vi "3_AdvancedDemo_HHT3.vi"() -> ()   [LabVIEW 2020]
uses:
  Types/HH_InputChannel.ctl
  Types/HH_UIThread_Cmds.ctl
  Types/HH_UIThread_Data.ctl
  _lib/PQ/HydraHarp/HH_InitInfo.ctl
  Types/HH_DataProcThread_QData.ctl
  Types/HH_DataProcThread_QCmds.ctl
  Types/HH_VisThread_QData.ctl
  Types/HH_VisThread_QCmds.ctl
  Types/HH_VisThread_Data.ctl
  _lib/PQ/HydraHarp/HH_RefSource.ctl
  _lib/PQ/HydraHarp/HH_MeasMode.ctl
  <vilib>/Utility/error.llb/DialogType.ctl
  _lib/PQ/HydraHarp/hhlib_x86_x64_UIThread.llb/HH_DllPath_global.vi
  <vilib>/Utility/error.llb/Error Cluster From Error Code.vi
  _lib/PQ/HydraHarp/HH_LibVersion_global.vi
  <vilib>/ErrorRing/Error Ring.xnode
panel:
  in  "Settings":bool=TRUE
  in  "Run continuously":bool caption="Conti."
  in  "Start":bool
  in  "Scale":bool
  out "CountRates":i32[](graph)
  in  "HistoAcqTime":dbl=1.0 caption="Int.Time    s" min=0.1 max=360000.0 step=0.1
  in  "AcqTime":i32=360000000 caption="T3Acq.   ms" min=1 max=360000 step=1
  in  "Binning":i32(ring) caption="Resol.      ps" items=["1", "2", "4", "8", "16", "32", "64", "128", "256", "512", "1024", "2048", "4096", "8192", "16384", "32768", "65536", "131072", "262144", "524288", "1048576", "2097152", "4194304", "8388608", "16777216", "33554432"]
  in  "HistoOffset":i32 caption="Offset      ns" min=0 max=500000 step=1
  out "DeltaT":dbl=inf caption="Resol.     ms" format="%.2f"
  in  "BitShift":i32=15 min=0 max=32 step=1
  in  "OvlLevel":i32=65536 caption="Ovl.Level" min=1024 max=65536 step=1024
  in  "StopOvl.":bool=TRUE
  out "TTraceGraph":T1(graph)
  out "HistoGraph":cluster{dbl, "Resol":dbl, "Histos":u32[][]}(graph)
  in  "SyncZeroX":i32=10 caption="ZeroCr.  mV" min=0 max=40 step=1
  in  "SyncDivider":i32(ring)=3 caption="Divider" items=["1", "2", "4", "8", "16"]
  in  "SyncOffset":i32 caption="Offset      ps" min=-99999 max=99999 step=1
  in  "SyncLevel":i32=50 caption="Level      mV" min=0 max=1000 step=1
  in  "Channels":T2[](array[typedef])=[{"Name"="Inp.Chan 1", "Enable"=TRUE, "Offset"=0, "CFDLevel"=50, "ZeroX"=10}, {"Name"="Inp.Chan 2", "Enable"=TRUE, "Offset"=0, "CFDLevel"=50, "ZeroX"=10}, {"Name"="Inp.Chan 3", "Enable"=TRUE, "Offset"=0, "CFDLevel"=50, "ZeroX"=10}, {"Name"="Inp.Chan 4", "Enable"=TRUE, "Offset"=0, "CFDLevel"=50, "ZeroX"=10}, {"Name"="Inp.Chan 5", "Enable"=TRUE, "Offset"=0, "CFDLevel"=50, "ZeroX"=10}, {"Name"="Inp.Chan 6", "Enable"=TRUE, "Offset"=0, "CFDLevel"=50, "ZeroX"=10}, {"Name"="Inp.Chan 7", "Enable"=TRUE, "Offset"=0, "CFDLevel"=50, "ZeroX"=10}, {"Name"="Inp.Chan 8", "Enable"=TRUE, "Offset"=0, "CFDLevel"=50, "ZeroX"=10}] {"ZeroX" min=0 max=40 step=1; "Offset" min=-99999 max=99999 step=1; "CFDLevel" min=0 max=1000 step=1}
  out "SyncRate":string="Sync Rate: 0 cps\n"
  out "OverRun":bool caption="Overrun:"
  out "Status":string="Elements in Q: 0"
  # "Histogram"
  # "Time Trace"
  # "Sync"
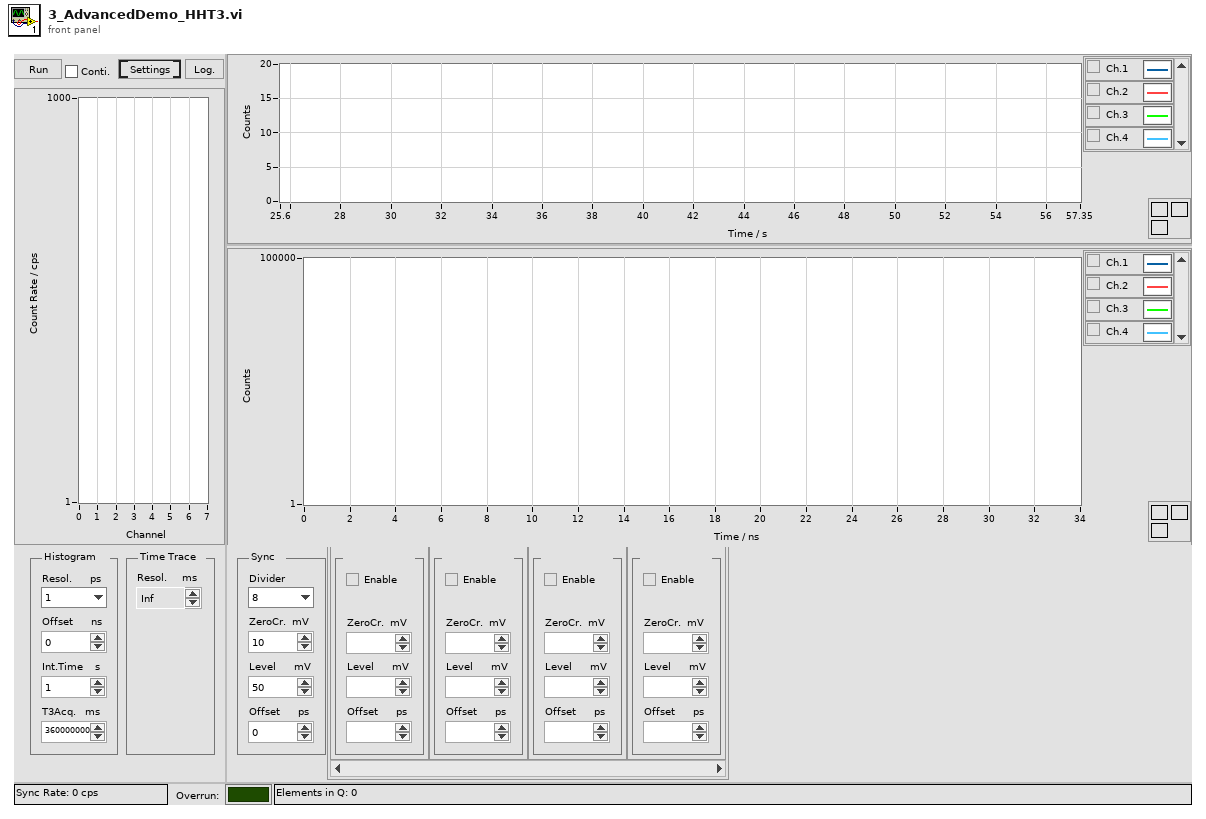
[diagram p1: front panel]
types:
  T1 = cluster{dbl, "Resolution":dbl, "Histogram":u32[][]}
  T2 = typedef "HH_InputChannel.ctl" = cluster{"Name":string, "Enable":bool, "Offset":i32, "CFDLevel":i32, "ZeroX":i32}
  T3 = typedef "HH_DataProcThread_QCmds.ctl" = enum16{"Exit", "Proc", "Init", "SetShift", "SetNumChannels", "SetHistAcqTime"}
  T4 = typedef "HH_VisThread_Data.ctl" = cluster{"Resol":dbl, "DeltaT":dbl, "NumChannels":i32}
  T5 = typedef "HH_VisThread_QData.ctl" = cluster{"Histos":u32[][], "Cmd":T6, "TimeTrace":u32[][], "Bin":i32, "Total bin":u64, "Status":string, "Resol":dbl, "DeltaT":dbl, "nChannels":i32}
  T6 = typedef "HH_VisThread_QCmds.ctl" = enum16{"_none_", "Resol", "nChannels", "DeltaT", "Histo", "TTrace", "Status"}
  T7 = typedef "HH_DataProcThread_QData.ctl" = cluster{"Cmd":T3, "nActual":i32, "Buffer":u32[], "TickCount":u32, "Param":i32}
  T8 = typedef "HH_UIThread_Data.ctl" = cluster{"Init Info":T9, "DevIdx":i32, "SyncDivider":i32, "SyncOffset":i32, "SyncLevel":i32, "Channels":T2[], "CurrentChannels":i32[], "AcqTime":i32, "Binning":i32, "HistoOffset":i32, "HistoLen":i32, "StopOvl.":bool, "OvlLevel":u32, "StartMeas":bool, "HistoLength":i32, "Resolution":dbl, "Run cont.":bool, "Status":string, "SyncRate":i32, "BitShift":i32, "HistoAcqTime":dbl, "SyncZeroX":i32, "SyncRateStart":i32}
  T9 = typedef "HH_InitInfo.ctl" = cluster{"Library Version":string, "Serial No.":string, "Model":string, "Partnum":string, "Version":string, "features":i32, "nchannels":i32, "nummod":i32, "Model Codes":i32[], "Version Codes":i32[], "Base Resolution":dbl, "Bin Steps":i32}
  T10 = typedef "HH_UIThread_Cmds.ctl" = enum16{"Idle", "Init", "SetInpChanEnable", "SetInpChanOffset", "SetInpChanTrg", "SetSyncDivider", "SetSyncTrg", "SetSyncOffset", "SetBinning", "SetHistoOffset", "SetHistoLen", "SetStopOvl", "SetBitShift", "SetHistoAcqTime", "GetRates", "StartMeas", "StopMeas", "AbortMeas", "GetResolution", "GetHisto", "ReadFiFo", "WriteStatus", "Resize", "EnableControls", "DisableControls", "Error", "Exit"}
  T11 = enum8{"Enabled", "Disabled", "Disabled and Grayed Out"}
  T12 = typedef "HH_MeasMode.ctl" = i32
  T13 = typedef "HH_RefSource.ctl" = enum16{"internal", "external"}
  T14 = typedef "DialogType.ctl" = u16
  T15 = cluster{"T0":dbl, "dt":dbl, "TimeTrace_out":u32[][]}
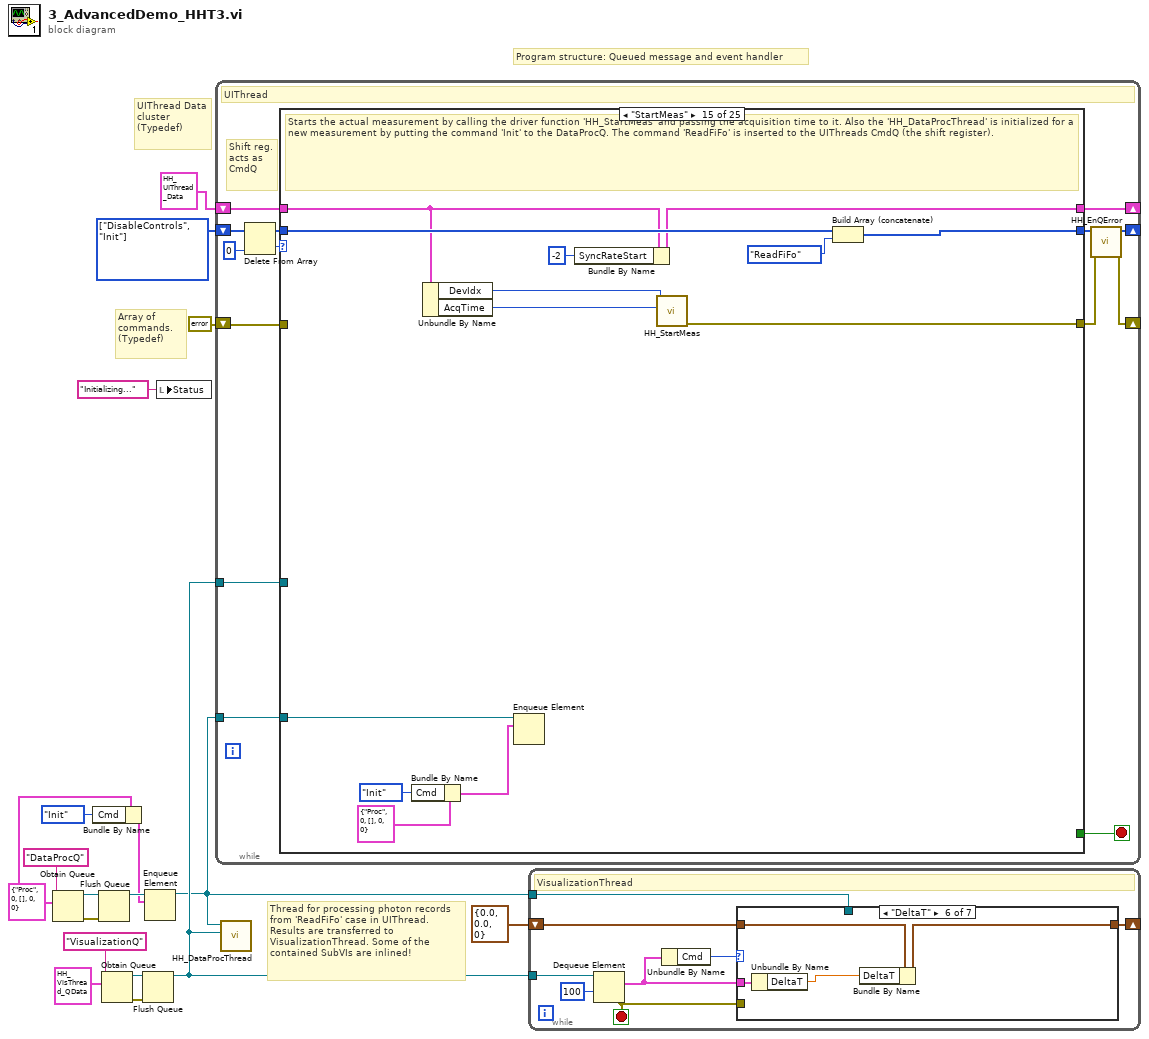
[diagram p0: block diagram]
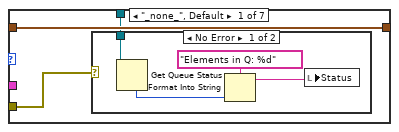
[diagram p2: hidden frame]
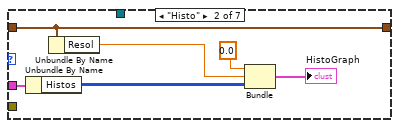
[diagram p4: hidden frame]
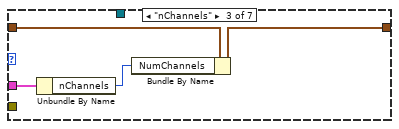
[diagram p5: hidden frame]
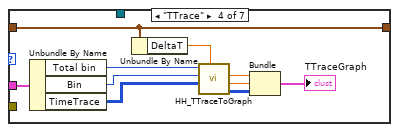
[diagram p6: hidden frame]
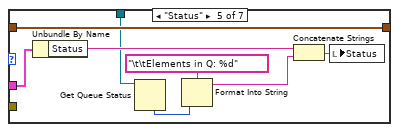
[diagram p7: hidden frame]
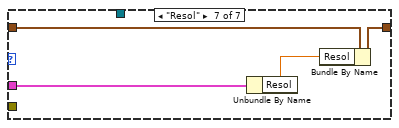
[diagram p8: hidden frame]
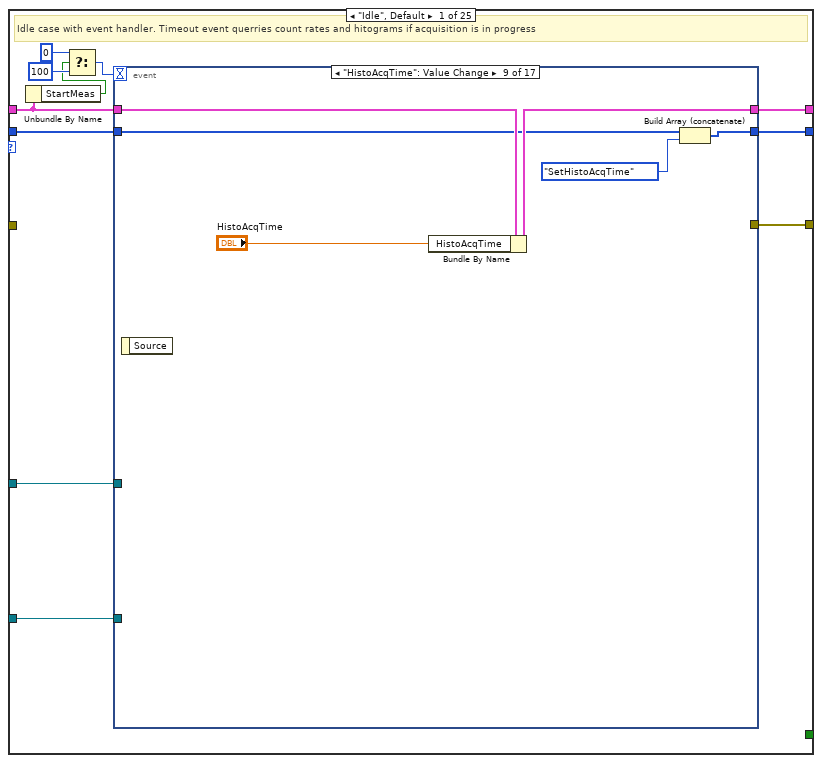
[diagram p9: hidden frame]
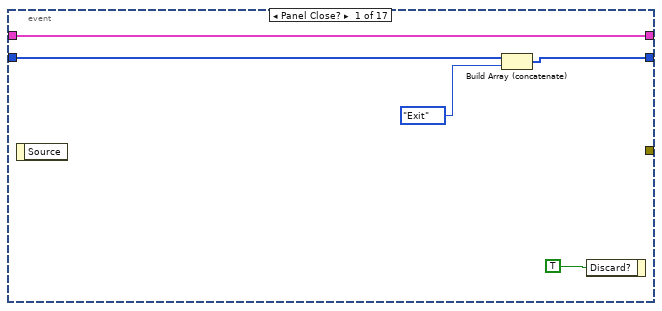
[diagram p10: hidden frame]
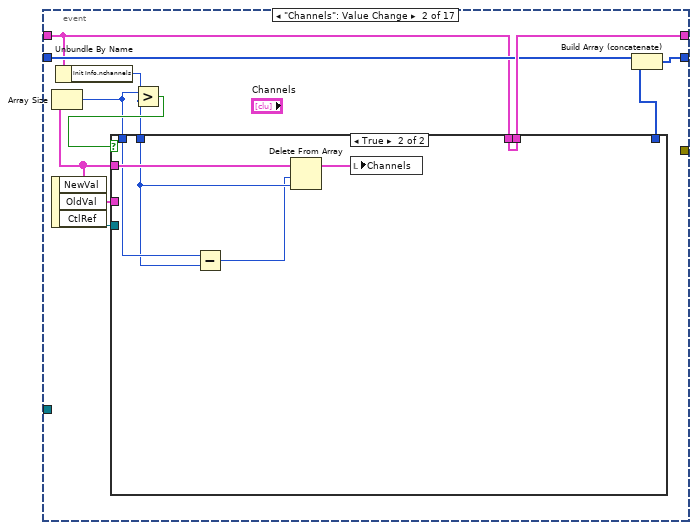
[diagram p11: hidden frame]
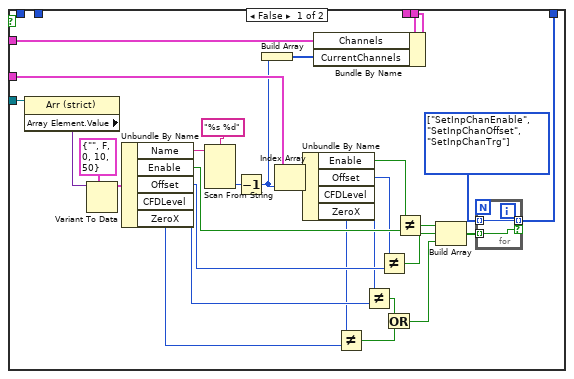
[diagram p12: hidden frame]
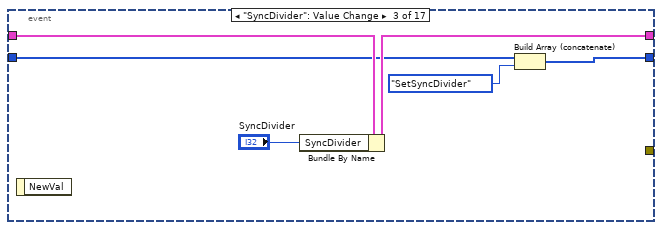
[diagram p13: hidden frame]
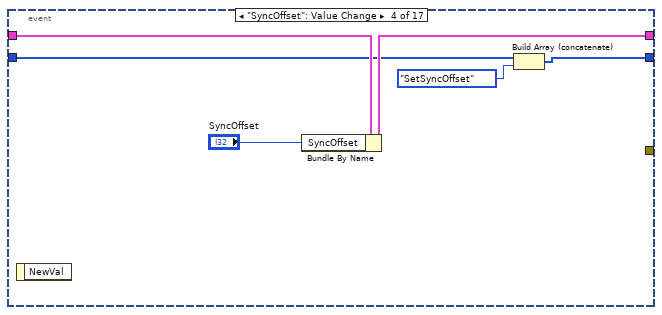
[diagram p14: hidden frame]
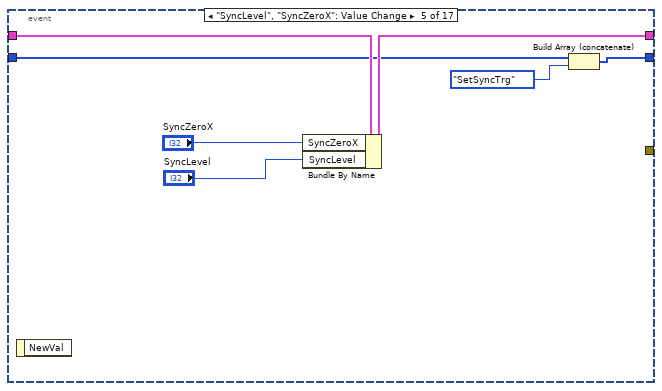
[diagram p15: hidden frame]
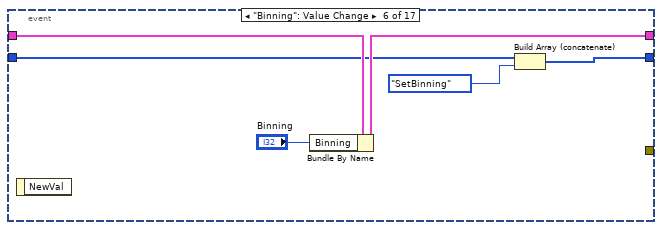
[diagram p16: hidden frame]
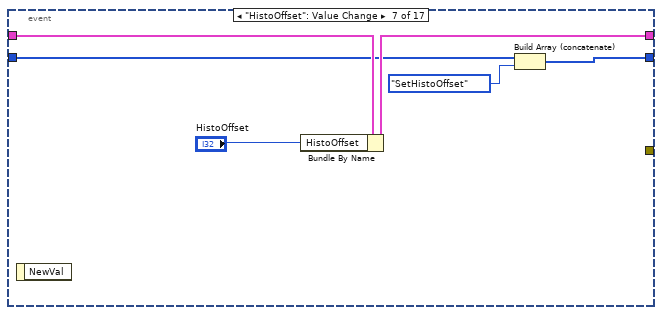
[diagram p17: hidden frame]
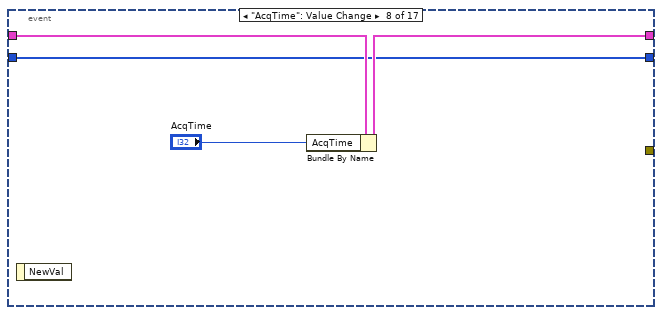
[diagram p18: hidden frame]
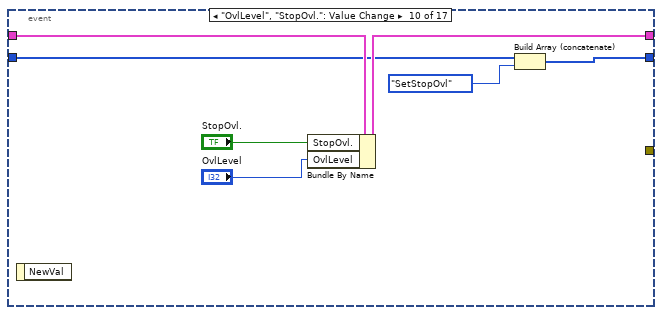
[diagram p19: hidden frame]
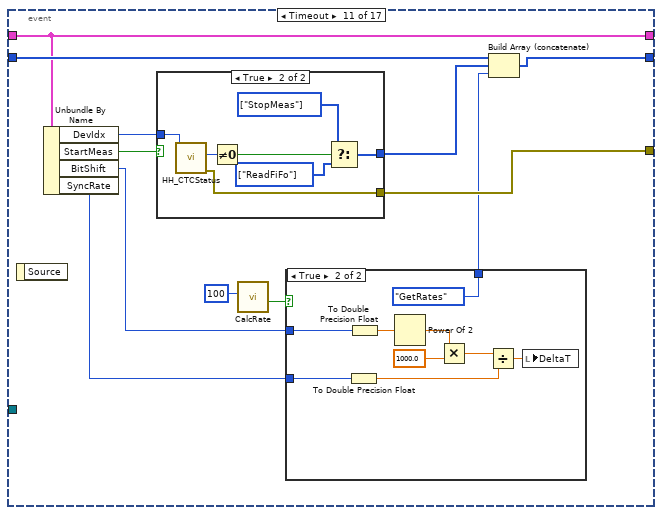
[diagram p20: hidden frame]
diagram:
  w4 = T7 {"Cmd"=enum."Proc", "nActual"=0, "Buffer"=[], "TickCount"=0, "Param"=0} ("MH_DataProcThread_QData")
  w17 = T10[] [enum."DisableControls", enum."Init"] items=["Idle", "Init", "SetInpChanEnable", "SetInpChanOffset", "SetInpChanTrg", "SetSyncDivider", "SetSyncTrg", "SetSyncOffset", "SetBinning", "SetHistoOffset", "SetHistoLen", "SetStopOvl", "SetBitShift", "SetHistoAcqTime", "GetRates", "StartMeas", "StopMeas", "AbortMeas", "GetResolution", "GetHisto", "ReadFiFo", "WriteStatus", "Resize", "EnableControls", "DisableControls", "Error", "Exit"]
  # "Thread for processing photon records from 'ReadFiFo' case in UIThread. Results are transferred to VisualizationThread. Some of the contained SubVIs are inlined!"
  # "Array of commands.\n(Typedef)"
  # "Program structure: Queued message and event handler"
  # "UIThread Data cluster\n(Typedef)"
  n1 = Obtain Queue(name (unnamed)="DataProcQ", element data type=w4) -> (queue out=w14:refnum<queue>, error out=w13:errorcluster)  [unwired: 3 in, 1 out]
  n2 = Bundle By Name(cluster=w4, "Cmd"=HH_DataProcThread_QCmds."Init") -> (w2:T7)
  n3 = Flush Queue(queue=w14, error in (no error)=w13) -> (queue out=w5:refnum<queue>)  [unwired: 2 out]
  n4 = Obtain Queue(name (unnamed)="VisualizationQ", element data type=T5 {"Histos"=[], "Cmd"=enum."_none_", "TimeTrace"=[], "Bin"=0, "Total bin"=0, "Status"="", "Resol"=0.0, "DeltaT"=0.0, "nChannels"=0} ("MH_GUIThread_QData")) -> (queue out=w12:refnum<queue>, error out=w11:errorcluster)  [unwired: 3 in, 1 out]
  n5 = Flush Queue(queue=w12, error in (no error)=w11) -> (queue out=w7:refnum<queue>)  [unwired: 2 out]
  n6 = Enqueue Element(queue=w5, element=w2) -> (queue out=w1:refnum<queue>)  [unwired: 2 in, 2 out]
  n7 = local write "Status"("Initializing..." ("Status")) -> ()
  n8 = while {
    shift-right: [w21] -> _
    shift-left: w17 -> [w28]
    shift-right: [w31] -> _
    shift-left: T8 {"Init Info"={"Library Version"="", "Serial No."="", "Model"="", "Partnum"="", "Version"="", "features"=0, "nchannels"=0, "nummod"=0, "Model Codes"=[], "Version Codes"=[], "Base Resolution"=0.0, "Bin Steps"=0}, "DevIdx"=0, "SyncDivider"=1, "SyncOffset"=0, "SyncLevel"=50, "Channels"=[], "CurrentChannels"=[], "AcqTime"=1, "Binning"=1, "HistoOffset"=1, "HistoLen"=1024, "StopOvl."=FALSE, "OvlLevel"=1024, "StartMeas"=FALSE, "HistoLength"=0, "Resolution"=0.0, "Run cont."=FALSE, "Status"="", "SyncRate"=0, "BitShift"=0, "HistoAcqTime"=0.0, "SyncZeroX"=10, "SyncRateStart"=0} -> [w30]
    shift-right: [w23] -> _
    shift-left: errorcluster {"status"=FALSE, "code"=0, "source"=""} ("error IO") -> [w29]
    tunnel: w1 -> [w20]
    tunnel: w7 -> [w19]
    stop <- w32 stop-if-true
    # "Shift reg.\nacts as\nCmdQ"
    # "UIThread"
    n9 = Delete From Array(array=w28, index=0) -> (deleted portion=w26:T10, array with subset deleted=w25:T10[])  [unwired: 1 in]
    n10 = case shown="\"StartMeas\"" w26 {
      tunnel: [w43 w272 w301 w315 w329 w346 w355 w357 w364 w372 w379 w399 w411 w420 w498 w503 w516 w533 w534 w560 w573 w580 w592 w598 w604] -> w22
      tunnel: [_ _ _ _ _ _ _ _ _ _ _ _ _ _ _ _ _ _ _ _ _ _ _ _ TRUE] -> w32
      tunnel: [w42 w253 w304 w318 w332 w348 w356 w361 w368 w373 w380 w384 w401 w423 w490 w506 w518 w529 w544 w559 w561 w579 w591 w599 w607] -> w31
      tunnel: w30 -> [w39 w258 w304 w318 w332 w348 w356 w361 w368 w373 w380 w384 w401 w419 w491 w507 w519 w530 w544 w559 w561 w579 w591 w599 w607]
      tunnel: [w40 w277 w302 w316 w330 w344 w354 w360 w367 w371 w378 _ _ w429 w501 w509 w521 w531 w539 _ _ _ _ _ w605] -> w24
      tunnel: w29 -> [_ _ _ _ _ _ _ _ _ _ _ _ _ _ _ _ _ _ _ _ _ _ _ w600 _]
      tunnel: w25 -> [w41 w274 w301 w315 w329 w346 w355 w357 w363 w372 w379 w399 w411 w421 w499 w504 w516 w533 w535 w560 w573 w580 w592 _ w604]
      tunnel: w20 -> [w34 w251 _ _ _ _ _ _ _ _ _ w385 w402 _ w495 _ _ _ w536 _ _ _ _ _ w603]
      tunnel: w19 -> [w33 w243 _ _ _ _ _ _ _ _ _ w386 _ _ _ _ _ w526 _ _ _ _ _ _ w602]
      frame "Idle", Default {
        # "Idle case with event handler. Timeout event querries count rates and hitograms if acquisition is in progress"
        n11 = Unbundle By Name(w39) -> ("StartMeas"=w37:bool)
        n12 = Select(t=0, s=w37, f=100) -> (s? t:f=w36:i32)
        n13 = event shown="[8] \"HistoAcqTime\": Value Change" {
          selector: _ -> [_ _ _ _ _ _ _ _ _ _ _ _ _ _ _ _ _]
          dyn-events: _ -> [_ _ _ _ _ _ _ _ _ _ _ _ _ _ _ _ _]
          timeout: w36 -> [_ _ _ _ _ _ _ _ _ _ _ _ _ _ _ _ _]
          tunnel: [w44 w54 w98 w104 w111 w118 w124 w129 w134 w141 w156 w174 w186 w204 w210 w218 w228] -> w43
          tunnel: [w47 w57 w102 w108 w115 w121 w127 w131 w137 w144 w155 w178 w185 w202 w209 w217 w231] -> w42
          tunnel: w39 -> [w47 w53 w103 w109 w116 w122 w128 w132 w138 w145 w155 w179 w183 w203 w209 w217 w231]
          tunnel: w41 -> [w46 w56 w100 w106 w113 w120 w126 w129 w135 w143 w157 w175 w187 w204 w210 w218 w229]
          tunnel: [_ _ _ _ _ _ _ _ _ _ w151 _ _ _ _ _ _] -> w40
          tunnel: w34 -> [_ _ _ _ _ _ _ _ _ _ _ _ _ _ _ _ _]
          tunnel: w33 -> [_ _ _ _ _ _ _ _ _ _ _ _ _ _ _ _ _]
          event Panel Close? {
            n14 = event-data() -> ()  [unwired: 1 in, 1 out]
            n15 = Build Array (concatenate)(w46, HH_UIThread_Cmds."Exit") -> (w44:T10[])
            n16 = event-data("Discard?"=TRUE) -> ()  [unwired: 1 in, 1 out]
          }
          event "Channels": Value Change {
            n17 = event-data() -> ("NewVal"=w52:T2[], "OldVal"=w58:T2[], "CtlRef"=w59:refnum<vi>)  [unwired: 1 in]
            n18 = Array Size(array=w52) -> (size(s)=w49:i32)
            n19 = Unbundle By Name(w53) -> ("Init Info.nchannels"=w50:i32)
            n20 = Greater?(x=w49, y=w50) -> (0:w51:bool)
            n21 = case shown="True" w51 {
              tunnel: w59 -> [w89 _]
              tunnel: w58 -> [w83 _]
              tunnel: [w66 w97] -> w57
              tunnel: [w64 _] -> w55
              tunnel: w53 -> [w61 w97]
              tunnel: w52 -> [w60 w96]
              tunnel: w50 -> [_ w94]
              tunnel: w49 -> [_ w95]
              frame False {
                w67 = T10[] [enum."SetInpChanEnable", enum."SetInpChanOffset", enum."SetInpChanTrg"] items=["Idle", "Init", "SetInpChanEnable", "SetInpChanOffset", "SetInpChanTrg", "SetSyncDivider", "SetSyncTrg", "SetSyncOffset", "SetBinning", "SetHistoOffset", "SetHistoLen", "SetStopOvl", "SetBitShift", "SetHistoAcqTime", "GetRates", "StartMeas", "StopMeas", "AbortMeas", "GetResolution", "GetHisto", "ReadFiFo", "WriteStatus", "Resize", "EnableControls", "DisableControls", "Error", "Exit"]
                n22 = property class="Arr (strict)"(reference=w89) -> ("Array Element.Value"=w88:variant)  [unwired: 1 in, 2 out]
                n23 = Variant To Data(type=T2 {"Name"="", "Enable"=FALSE, "Offset"=0, "CFDLevel"=10, "ZeroX"=50} ("Channel"), Variant=w88) -> (data=w65:T2)  [unwired: 1 in, 1 out]
                n24 = Unbundle By Name(w65) -> ("Name"=w86:string, "Enable"=w80:bool, "Offset"=w78:i32, "CFDLevel"=w76:i32, "ZeroX"=w74:i32)
                n25 = Scan From String(format string="%s %d", input string=w86) -> (output 2=w84:i32)  [unwired: 5 in, 3 out]
                n26 = Decrement(x=w84) -> (x-1=w63:i32)
                n27 = Build Array(w63) -> (w62:i32[])
                n28 = Index Array(array=w83, index=w63) -> (element=w82:T2)
                n29 = Unbundle By Name(w82) -> ("Enable"=w81:bool, "Offset"=w79:i32, "CFDLevel"=w77:i32, "ZeroX"=w75:i32)
                n30 = Bundle By Name(cluster=w61, "Channels"=w60, "CurrentChannels"=w62) -> (w66:T8)
                n31 = Not Equal?(x=w75, y=w74) -> (x != y?=w69:bool)
                n32 = Not Equal?(x=w77, y=w76) -> (x != y?=w70:bool)
                n33 = Not Equal?(x=w79, y=w78) -> (x != y?=w72:bool)
                n34 = Or(x=w70, y=w69) -> (x .or. y?=w68:bool)
                n35 = Not Equal?(x=w81, y=w80) -> (x != y?=w73:bool)
                n36 = Build Array(w73, w72, w68) -> (w71:bool[])
                n37 = for {
                  tunnel: w71 -> [w90] mode=indexing
                  tunnel: w67 -> [w91] mode=indexing
                  tunnel: [w91] -> w64 mode=indexing if=w90
                }
              }
              frame True {
                n38 = Subtract(x=w95, y=w94) -> (x-y=w93:i32)
                n39 = Delete From Array(array=w96, length=w93, index=w94) -> (array with subset deleted=w92:T2[])  [unwired: 1 out]
                n40 = local write "Channels"(w92) -> ()
              }
            }
            n41 = Build Array (concatenate)(w56, w55) -> (w54:T10[])
          }
          event "SyncDivider": Value Change {
            n42 = event-data() -> ()  [unwired: 1 in, 1 out]
            n43 = Bundle By Name(cluster=w103, "SyncDivider"="SyncDivider") -> (w102:T8)
            n44 = Build Array (concatenate)(w100, HH_UIThread_Cmds."SetSyncDivider") -> (w98:T10[])
          }
          event "SyncOffset": Value Change {
            n45 = event-data() -> ()  [unwired: 1 in, 1 out]
            n46 = Bundle By Name(cluster=w109, "SyncOffset"="SyncOffset") -> (w108:T8)
            n47 = Build Array (concatenate)(w106, HH_UIThread_Cmds."SetSyncOffset") -> (w104:T10[])
          }
          event "SyncLevel", "SyncZeroX": Value Change {
            n48 = event-data() -> ()  [unwired: 1 in, 1 out]
            n49 = Bundle By Name(cluster=w116, "SyncZeroX"="SyncZeroX", "SyncLevel"="SyncLevel") -> (w115:T8)
            n50 = Build Array (concatenate)(w113, HH_UIThread_Cmds."SetSyncTrg") -> (w111:T10[])
          }
          event "Binning": Value Change {
            n51 = event-data() -> ()  [unwired: 1 in, 1 out]
            n52 = Bundle By Name(cluster=w122, "Binning"="Binning") -> (w121:T8)
            n53 = Build Array (concatenate)(w120, HH_UIThread_Cmds."SetBinning") -> (w118:T10[])
          }
          event "HistoOffset": Value Change {
            n54 = event-data() -> ()  [unwired: 1 in, 1 out]
            n55 = Bundle By Name(cluster=w128, "HistoOffset"="HistoOffset") -> (w127:T8)
            n56 = Build Array (concatenate)(w126, HH_UIThread_Cmds."SetHistoOffset") -> (w124:T10[])
          }
          event "AcqTime": Value Change {
            n57 = event-data() -> ()  [unwired: 1 in, 1 out]
            n58 = Bundle By Name(cluster=w132, "AcqTime"="AcqTime") -> (w131:T8)
          }
          event "HistoAcqTime": Value Change {
            n59 = event-data() -> ()  [unwired: 1 in, 1 out]
            n60 = Bundle By Name(cluster=w138, "HistoAcqTime"="HistoAcqTime") -> (w137:T8)
            n61 = Build Array (concatenate)(w135, HH_UIThread_Cmds."SetHistoAcqTime") -> (w134:T10[])
          }
          event "OvlLevel", "StopOvl.": Value Change {
            n62 = event-data() -> ()  [unwired: 1 in, 1 out]
            n63 = Bundle By Name(cluster=w145, "StopOvl."="StopOvl.", "OvlLevel"="OvlLevel") -> (w144:T8)
            n64 = Build Array (concatenate)(w143, HH_UIThread_Cmds."SetStopOvl") -> (w141:T10[])
          }
          event Timeout {
            n65 = event-data() -> ()  [unwired: 1 in, 1 out]
            n66 = Unbundle By Name(w155) -> ("DevIdx"=w153:i32, "StartMeas"=w154:bool, "BitShift"=w150:i32, "SyncRate"=w149:i32)
            n67 = case shown="True" w154 {
              tunnel: w153 -> [_ w173]
              tunnel: [_ w171] -> w152
              tunnel: [_ w168] -> w151
              frame False {
              }
              frame True {
                w169 = T10[] [enum."ReadFiFo"] items=["Idle", "Init", "SetInpChanEnable", "SetInpChanOffset", "SetInpChanTrg", "SetSyncDivider", "SetSyncTrg", "SetSyncOffset", "SetBinning", "SetHistoOffset", "SetHistoLen", "SetStopOvl", "SetBitShift", "SetHistoAcqTime", "GetRates", "StartMeas", "StopMeas", "AbortMeas", "GetResolution", "GetHisto", "ReadFiFo", "WriteStatus", "Resize", "EnableControls", "DisableControls", "Error", "Exit"]
                w170 = T10[] [enum."StopMeas"] items=["Idle", "Init", "SetInpChanEnable", "SetInpChanOffset", "SetInpChanTrg", "SetSyncDivider", "SetSyncTrg", "SetSyncOffset", "SetBinning", "SetHistoOffset", "SetHistoLen", "SetStopOvl", "SetBitShift", "SetHistoAcqTime", "GetRates", "StartMeas", "StopMeas", "AbortMeas", "GetResolution", "GetHisto", "ReadFiFo", "WriteStatus", "Resize", "EnableControls", "DisableControls", "Error", "Exit"]
                n68 = call "HH_CTCStatus.vi"("devidx"=w173) -> ("error out"=w168:errorcluster, "ctcstatus"=w172:i32)  [unwired: 8 in, 1 out]
                n69 = Not Equal To 0?(x=w172) -> (x != 0?=w167:bool)
                n70 = Select(t=w170, s=w167, f=w169) -> (s? t:f=w171:T10[])
              }
            }
            n71 = call "CalcRate.vi"("Refresh(ms)"=u32 100) -> ("updated?"=w147:bool)  [unwired: 8 in, 2 out]
            n72 = case shown="True" w147 {
              tunnel: w150 -> [_ w160]
              tunnel: w149 -> [_ w159]
              tunnel: [_ HH_UIThread_Cmds."GetRates"] -> w148
              frame False {
              }
              frame True {
                n73 = To Double Precision Float(number=w159) -> (double precision float=w164:dbl)
                n74 = To Double Precision Float(number=w160) -> (double precision float=w165:dbl)
                n75 = Power Of 2(x=w165) -> (2^x=w163:dbl)
                n76 = Multiply(x=w163, y=1000.0) -> (x*y=w162:dbl)
                n77 = Divide(x=w162, y=w164) -> (x/y=w166:dbl)
                n78 = local write "DeltaT"(w166) -> ()
              }
            }
            n79 = Build Array (concatenate)(w157, w152, w148) -> (w156:T10[])
          }
          event "BitShift": Value Change {
            n80 = event-data() -> ()  [unwired: 1 in, 1 out]
            n81 = Bundle By Name(cluster=w179, "BitShift"="BitShift") -> (w178:T8)
            n82 = Build Array (concatenate)(w175, HH_UIThread_Cmds."SetBitShift") -> (w174:T10[])
          }
          event "Start": Value Change {
            n83 = event-data() -> ()  [unwired: 1 in, 1 out]
            n84 = Unbundle By Name(w183) -> ("SyncRate"=w182:i32)
            n85 = Greater Or Equal?(x=w182, y=10) -> (x >= y?=w180:bool)
            n86 = case shown="True" w180 {
              selector: w180 -> [w189 _]
              tunnel: w187 -> [w191 w200]
              tunnel: [w191 w198] -> w186
              tunnel: [w190 w197] -> w185
              tunnel: "Start" -> [_ w196]
              tunnel: w183 -> [w190 w192]
              frame False {
                n87 = local write "Start"(w189) -> ()
                n88 = One Button Dialog(message="SyncRate too low!!!" ("Status")) -> ()  [unwired: 1 in, 1 out]
              }
              frame True {
                w195 = T10[] [enum."SetBitShift", enum."SetHistoAcqTime", enum."StartMeas"] items=["Idle", "Init", "SetInpChanEnable", "SetInpChanOffset", "SetInpChanTrg", "SetSyncDivider", "SetSyncTrg", "SetSyncOffset", "SetBinning", "SetHistoOffset", "SetHistoLen", "SetStopOvl", "SetBitShift", "SetHistoAcqTime", "GetRates", "StartMeas", "StopMeas", "AbortMeas", "GetResolution", "GetHisto", "ReadFiFo", "WriteStatus", "Resize", "EnableControls", "DisableControls", "Error", "Exit"]
                # "When starting a measurement three commands are added to the CmdQ (the shift register) and get processed in the corresponding cases of the UIThread: \n\n1. 'SetBitShift': Parameter determining the  temporal resolution of the photons time trace\n\n2. 'SetHistoAcqTime': The time interval for accumulating a histogram from the photon stream (for details refer to the corresponding case)\n\n3. 'StartMeas': Starts the actual measurement (for details refer to the corresponding case)"
                n89 = Bundle By Name(cluster=w192, "StartMeas"=w196) -> (w197:T8)
                n90 = Build Array(HH_UIThread_Cmds."AbortMeas") -> (w193:T10[])
                n91 = Select(t=w195, s=w196, f=w193) -> (s? t:f=w199:T10[])
                n92 = Build Array (concatenate)(w200, w199) -> (w198:T10[])
              }
            }
          }
          event "Run continuously": Value Change {
            n93 = event-data() -> ()  [unwired: 1 in, 1 out]
            n94 = Bundle By Name(cluster=w203, "Run cont."="Run continuously") -> (w202:T8)
          }
          event "Scale": Value Change {
            n95 = event-data() -> ()  [unwired: 1 in, 1 out]
            n96 = Select(t=u8 0 ("Y Scale.Mapping Mode"), s="Scale", f=u8 1 ("Y Scale.Mapping Mode")) -> (s? t:f=w205:u8)
            n97 = property on="HistoGraph" class="WFGraph (strict)"("YScale.Mapping Mode"=w205) -> ()  [unwired: 2 in, 2 out]
          }
          event "Settings": Value Change {
            n98 = event-data() -> ()  [unwired: 1 in, 1 out]
            n99 = property on="Splitter" class="Splitter"() -> ("Position"=w216:i32)  [unwired: 2 in, 2 out]
            n100 = Select(t=237 ("PosT"), s="Settings", f=0 ("PosF")) -> (s? t:f=w213:i32)
            n101 = Subtract(x=w216, y=w213) -> (x-y=w212:i32)
            n102 = while {
              shift-right: [w227] -> _
              shift-left: w212 -> [w220]
              i -> [w226]
              stop <- w223 stop-if-true
              n103 = property on="Splitter 4" class="Splitter"("Position"=w220) -> (error out=w219:errorcluster)  [unwired: 2 in, 1 out]
              n104 = Greater Or Equal?(x=w226, y=10) -> (x >= y?=w224:bool)
              n105 = Decrement(x=w220) -> (x-1=w227:i32)
              n106 = Unbundle(w219) -> ("status"=w222:bool)  [unwired: 2 out]
              n107 = Not(x=w222) -> (.not. x?=w221:bool)
              n108 = Or(x=w221, y=w224) -> (x .or. y?=w223:bool)
            }
          }
          event Panel Resize {
            n109 = event-data() -> ()  [unwired: 1 in, 1 out]
            n110 = Build Array (concatenate)(w229, HH_UIThread_Cmds."Resize") -> (w228:T10[])
          }
        }
      }
      frame "Init" {
        w234 = T12 3 items=["Histo"=0, "T2"=2, "T3"=3, "Conti"=8]  # mode
        w233 = HH_RefSource."internal"  # refsource
        w241 = 1.0 ("HistoAcqTime")
        w242 = 15 ("Value (Signaling)")
        w260 = FALSE ("Run cont.")
        w262 = FALSE ("StartMeas")
        w263 = 65536 ("OvlLevel")
        w264 = TRUE ("StopOvl.")
        w265 = 360000000 ("AcqTime")
        w266 = 0 ("HistoOffset")
        w267 = 0 ("Binning")
        w268 = 50 ("SyncLevel")
        w269 = 10 ("SyncZeroX")
        w270 = 0 ("SyncOffset")
        w271 = 3 ("SyncDivider")
        w273 = T10[] [enum."SetSyncDivider", enum."SetSyncOffset", enum."SetSyncTrg", enum."SetInpChanEnable", enum."SetInpChanOffset", enum."SetInpChanTrg", enum."SetBinning", enum."SetHistoOffset", enum."Resize", enum."EnableControls", enum."GetRates", enum."SetBitShift", enum."SetHistoAcqTime", enum."WriteStatus"] items=["Idle", "Init", "SetInpChanEnable", "SetInpChanOffset", "SetInpChanTrg", "SetSyncDivider", "SetSyncTrg", "SetSyncOffset", "SetBinning", "SetHistoOffset", "SetHistoLen", "SetStopOvl", "SetBitShift", "SetHistoAcqTime", "GetRates", "StartMeas", "StopMeas", "AbortMeas", "GetResolution", "GetHisto", "ReadFiFo", "WriteStatus", "Resize", "EnableControls", "DisableControls", "Error", "Exit"]
        # "100 x 60 x 60 x 1000 = 100 h"
        # "Init all FP controls and corresponding copy in UIThread Data cluster"
        # "EnQ list of commands"
        # "Array with Inp.Chan."
        # "Initialization: 1. Init HW -> get # of channels -> make array for Inp.Channels\n2. Init all FP controls and corresponding fields in UIThread Data cluster\n3. EnQ list of commands for further initialization"
        n111 = xnode "Error Ring"() -> ("error out"=w235:errorcluster)
        n112 = call "GetDLLPath.vi"("DllName_32bit"="HHLib.dll" ("name or relative path"), "DllName_64bit"="HHLib64.dll" ("name or relative path")) -> ("file exists?"=w237:bool, "DLLPath"=w238:path)  [unwired: 8 in]
        n113 = global write "HH_DllPath_global.vi" "DllPath"(w238) -> ()
        n114 = Select(t=errorcluster {"status"=FALSE, "code"=0, "source"=""} ("error IO"), s=w237, f=w235) -> (s? t:f=w254:errorcluster)
        n115 = global read "HH_LibVersion_global.vi" "Library Version"() -> (w232:string)
        n116 = Build Array (concatenate)(w274, w273) -> (w272:T10[])
        n117 = call "InitHH_UIThread.vi"("error in (no error)"=w254, "mode"=w234, "refsource"=w233, "Library Version"=w232) -> ("error out"=w277:errorcluster, "Init Info"=w280:T9, "DevIdx"=w279:i32)  [unwired: 5 in]
        n118 = local write "SyncDivider"(w271) -> ()
        n119 = local write "SyncOffset"(w270) -> ()
        n120 = local write "SyncZeroX"(w269) -> ()
        n121 = local write "SyncLevel"(w268) -> ()
        n122 = local write "Binning"(w267) -> ()
        n123 = local write "HistoOffset"(w266) -> ()
        n124 = Bundle By Name(cluster=w258, "DevIdx"=w279, "Init Info"=w280, "Status"="Initialized!") -> (w257:T8)
        n125 = Unbundle By Name(w257) -> ("Init Info.Bin Steps"=w256:i32, "Init Info.nchannels"=w244:i32)
        n126 = for {
          N: w244 -> [_]
          tunnel: T2 {"Name"="", "Enable"=FALSE, "Offset"=0, "CFDLevel"=10, "ZeroX"=50} ("Channel") -> [w297]
          tunnel: [w296] -> w276 mode=indexing
          tunnel: [w286] -> w275 mode=indexing
          i -> [w286]
          # "Init values for Inp. Channels"
          n127 = Increment(x=w286) -> (x+1=w289:i32)
          n128 = Format Into String(format string="Inp.Chan %d", w289) -> (resulting string=w294:string)  [unwired: 2 in, 1 out]
          n129 = Format Into String(format string="Ch.%d", w289) -> (resulting string=w287:string)  [unwired: 2 in, 1 out]
          n130 = Bundle By Name(cluster=w297, "Name"=w294, "Enable"=TRUE, "Offset"=0, "CFDLevel"=50 ("CFDZeroX"), "ZeroX"=10 ("CFDLevel")) -> (w296:T2)
          n131 = property on="HistoGraph" class="WFGraph (strict)"("Active Plot"=w286, "Plot.Plot Name"=w287) -> ()  [unwired: 2 in, 2 out]
          n132 = property on="TTraceGraph" class="WFGraph (strict)"("Active Plot"=w286, "Plot.Plot Name"=w287) -> ()  [unwired: 2 in, 2 out]
        }
        n133 = Bundle By Name(cluster=T5 {"Histos"=[], "Cmd"=enum."_none_", "TimeTrace"=[], "Bin"=0, "Total bin"=0, "Status"="", "Resol"=0.0, "DeltaT"=0.0, "nChannels"=0} ("MH_GUIThread_QData"), "Cmd"=HH_VisThread_QCmds."nChannels", "nChannels"=w244) -> (w246:T5)
        n134 = call "HH_CalcBinningValues.vi"("Bin Steps"=w256) -> ("BinningValues"=w261:cluster{"String":string, "Value":i32}[])  [unwired: 10 in]
        n135 = property on="Binning" class="Ring (strict)"("StringsAndValues[]"=w261) -> ()  [unwired: 2 in, 2 out]
        n136 = Bundle By Name(cluster=T7 {"Cmd"=enum."Proc", "nActual"=0, "Buffer"=[], "TickCount"=0, "Param"=0} ("MH_DataProcThread_QData"), "Param"=w244, "Cmd"=HH_DataProcThread_QCmds."SetNumChannels") -> (w250:T7)
        n137 = Enqueue Element(queue=w243, element=w246) -> ()  [unwired: 2 in, 3 out]
        n138 = Enqueue Element(queue=w251, element=w250) -> ()  [unwired: 2 in, 3 out]
        n139 = local write "Channels"(w276) -> ()
        n140 = Bundle By Name(cluster=w257, "Channels"=w276, "CurrentChannels"=w275, "SyncDivider"=w271, "SyncOffset"=w270, "SyncZeroX"=w269, "SyncLevel"=w268, "Binning"=w267, "HistoOffset"=w266, "AcqTime"=w265, "StopOvl."=w264, "OvlLevel"=w263, "StartMeas"=w262, "Run cont."=w260, "BitShift"=w242, "HistoAcqTime"=w241) -> (w253:T8)
        n141 = local write "StopOvl."(w264) -> ()
        n142 = local write "OvlLevel"(w263) -> ()
        n143 = local write "Start"(w262) -> ()
        n144 = local write "Run continuously"(w260) -> ()
        n145 = local write "BitShift"(w242) -> ()
        n146 = local write "AcqTime"(w265) -> ()
        n147 = local write "HistoAcqTime"(w241) -> ()
        n148 = property on="Settings" class="Bool (strict)"("Val(Sgnl)"=TRUE ("Value (Signaling)")) -> ()  [unwired: 2 in, 2 out]
        n149 = property on="Scale" class="Bool (strict)"("Val(Sgnl)"=FALSE ("Value (Signaling)")) -> ()  [unwired: 2 in, 2 out]
      }
      frame "SetInpChanEnable" {
        n150 = Unbundle By Name(w304) -> ("DevIdx"=w303:i32, "Channels"=w298:T2[], "CurrentChannels"=w299:i32[])
        n151 = for {
          tunnel: w303 -> [w311]
          shift-right: [w310] -> w302
          shift-left: errorcluster {"status"=FALSE, "code"=0, "source"=""} ("error out") -> [w309]
          tunnel: w299 -> [w305] mode=indexing
          tunnel: w298 -> [w308]
          n152 = Index Array(array=w308, index=w305) -> (element=w307:T2)
          n153 = Unbundle By Name(w307) -> ("Enable"=w306:bool)
          n154 = call "HH_SetInputChannelEnable.vi"("error in (no error)"=w309, "enable"=w306, "channel"=w305, "devidx"=w311) -> ("error out"=w310:errorcluster)  [unwired: 6 in, 1 out]
        }
      }
      frame "SetInpChanOffset" {
        n155 = Unbundle By Name(w318) -> ("DevIdx"=w317:i32, "Channels"=w312:T2[], "CurrentChannels"=w313:i32[])
        n156 = for {
          tunnel: w317 -> [w323]
          shift-right: [w320] -> w316
          shift-left: errorcluster {"status"=FALSE, "code"=0, "source"=""} ("error out") -> [w321]
          tunnel: w313 -> [w322] mode=indexing
          tunnel: w312 -> [w325]
          n157 = Index Array(array=w325, index=w322) -> (element=w324:T2)
          n158 = Unbundle By Name(w324) -> ("Offset"=w319:i32)
          n159 = call "HH_SetInputChannelOffset.vi"("error in (no error)"=w321, "Offset"=w319, "channel"=w322, "devidx"=w323) -> ("error out"=w320:errorcluster)  [unwired: 6 in, 1 out]
        }
      }
      frame "SetInpChanTrg" {
        n160 = Unbundle By Name(w332) -> ("DevIdx"=w331:i32, "Channels"=w326:T2[], "CurrentChannels"=w327:i32[])
        n161 = for {
          tunnel: w331 -> [w335]
          shift-right: [w337] -> w330
          shift-left: errorcluster {"status"=FALSE, "code"=0, "source"=""} ("error out") -> [w338]
          tunnel: w327 -> [w336] mode=indexing
          tunnel: w326 -> [w340]
          n162 = Index Array(array=w340, index=w336) -> (element=w339:T2)
          n163 = Unbundle By Name(w339) -> ("CFDLevel"=w334:i32, "ZeroX"=w333:i32)
          n164 = call "HH_SetInputCFD.vi"("CFD Channel"=w336, "error in (no error)"=w338, "CFD ZeroCross"=w333, "CFD Level"=w334, "devidx"=w335) -> ("error out"=w337:errorcluster)  [unwired: 5 in, 1 out]
        }
      }
      frame "SetSyncDivider" {
        n165 = Unbundle By Name(w348) -> ("DevIdx"=w347:i32, "SyncDivider"=w343:i32)
        n166 = Power Of 2(x=w343) -> (2^x=w342:dbl)
        n167 = To Long Integer(number=w342) -> (32bit integer=w341:i32)
        n168 = call "HH_SetSyncDiv.vi"("SyncDivider"=w341, "devidx"=w347) -> ("error out"=w345:errorcluster)  [unwired: 8 in, 1 out]
        n169 = flat-sequence {
          tunnel: w345 -> [w349]
          tunnel: [w349] -> w344
          frame #0 {
            n170 = Wait (ms)(milliseconds to wait=u32 100) -> ()  [unwired: 1 out]
          }
        }
      }
      frame "SetSyncTrg" {
        n171 = Unbundle By Name(w356) -> ("DevIdx"=w353:i32, "SyncLevel"=w351:i32, "SyncZeroX"=w352:i32)
        n172 = call "HH_SetSyncCFD.vi"("CFD ZeroCross"=w352, "CFD Level"=w351, "devidx"=w353) -> ("error out"=w354:errorcluster)  [unwired: 7 in, 1 out]
      }
      frame "SetSyncOffset" {
        n173 = Unbundle By Name(w361) -> ("DevIdx"=w359:i32, "SyncOffset"=w358:i32)
        n174 = call "HH_SetSyncChannelOffset.vi"("Offset"=w358, "devidx"=w359) -> ("error out"=w360:errorcluster)  [unwired: 8 in, 1 out]
      }
      frame "SetBinning" {
        # "When binning is changed the new resolution is querried"
        n175 = Unbundle By Name(w368) -> ("DevIdx"=w366:i32, "Binning"=w365:i32)
        n176 = call "HH_SetBinning.vi"("Binning"=w365, "devidx"=w366) -> ("error out"=w367:errorcluster)  [unwired: 8 in, 1 out]
        n177 = Build Array (concatenate)(HH_UIThread_Cmds."GetResolution", w363) -> (w364:T10[])
      }
      frame "SetHistoOffset" {
        n178 = Unbundle By Name(w373) -> ("DevIdx"=w370:i32, "HistoOffset"=w369:i32)
        n179 = call "HH_SetOffset.vi"("Offset"=w369, "devidx"=w370) -> ("error out"=w371:errorcluster)  [unwired: 8 in, 1 out]
      }
      frame "SetStopOvl" {
        n180 = Unbundle By Name(w380) -> ("DevIdx"=w377:i32, "StopOvl."=w376:bool, "OvlLevel"=w375:u32)
        n181 = To Unsigned Long Integer(number=w375) -> (unsigned 32bit integer=w374:u32)
        n182 = call "HH_SetStopOverflow.vi"("stopcount"=w374, "StopOnOverflow"=w376, "devidx"=w377) -> ("error out"=w378:errorcluster)  [unwired: 7 in, 1 out]
      }
      frame "SetBitShift" {
        n183 = Unbundle By Name(w384) -> ("BitShift"=w382:i32, "SyncRate"=w383:i32)
        n184 = Negate(x=w382) -> (-x=w392:i32)
        n185 = Bundle By Name(cluster=T7 {"Cmd"=enum."Proc", "nActual"=0, "Buffer"=[], "TickCount"=0, "Param"=0} ("MH_DataProcThread_QData"), "Param"=w392, "Cmd"=HH_DataProcThread_QCmds."SetShift") -> (w398:T7)
        n186 = To Double Precision Float(number=w382) -> (double precision float=w397:dbl)
        n187 = To Double Precision Float(number=w383) -> (double precision float=w396:dbl)
        n188 = Power Of 2(x=w397) -> (2^x=w395:dbl)
        n189 = Enqueue Element(queue=w385, element=w398) -> ()  [unwired: 2 in, 3 out]
        n190 = Multiply(x=w395, y=1000.0) -> (x*y=w394:dbl)
        n191 = Divide(x=w394, y=w396) -> (x/y=w381:dbl)
        "DeltaT" <- w381
        n192 = Bundle By Name(cluster=T5 {"Histos"=[], "Cmd"=enum."_none_", "TimeTrace"=[], "Bin"=0, "Total bin"=0, "Status"="", "Resol"=0.0, "DeltaT"=0.0, "nChannels"=0} ("MH_GUIThread_QData"), "DeltaT"=w381, "Cmd"=HH_VisThread_QCmds."DeltaT") -> (w393:T5)
        n193 = Enqueue Element(queue=w386, element=w393) -> ()  [unwired: 2 in, 3 out]
      }
      frame "SetHistoAcqTime" {
        # "The time interval for accumulating a histogram from the photon stream is set on the front panel by the control labeled 'Int.Time  [s]' and saved to the UIThread Data cluster in the variable 'HistoAcqTime' (refer to case 'Idle' -> EventCase \"HistoAcqTime\": Value Change). Knowing the  SyncRate, from 'HistoAcqTime' the number of Sync-Pulses that would occur during that time intervall are calculated here and are send to 'HH_DataProcThread' by putting this number to 'Param' together with the command 'SetHistAcqTime' in the DataProcQ."
        n194 = Unbundle By Name(w401) -> ("SyncRate"=w407:i32, "HistoAcqTime"=w400:dbl)
        n195 = To Double Precision Float(number=w407) -> (double precision float=w410:dbl)
        n196 = Multiply(x=w410, y=w400) -> (x*y=w409:dbl)
        n197 = Round To Nearest(number=w409) -> (nearest integer value=w408:dbl)
        n198 = To Long Integer(number=w408) -> (32bit integer=w406:i32)
        n199 = Bundle By Name(cluster=T7 {"Cmd"=enum."Proc", "nActual"=0, "Buffer"=[], "TickCount"=0, "Param"=0} ("MH_DataProcThread_QData"), "Param"=w406, "Cmd"=HH_DataProcThread_QCmds."SetHistAcqTime") -> (w405:T7)
        n200 = Enqueue Element(queue=w402, element=w405) -> ()  [unwired: 2 in, 3 out]
      }
      frame "GetRates" {
        n201 = Unbundle By Name(w419) -> ("Init Info.nchannels"=w428:i32, "Channels"=w424:T2[], "DevIdx"=w415:i32, "StartMeas"=w422:bool, "SyncRateStart"=w413:i32)  [unwired: 1 out]
        n202 = call "HH_GetSyncRate.vi"("devidx"=w415) -> ("error out"=w417:errorcluster, "syncrate"=w414:i32)  [unwired: 8 in, 1 out]
        n203 = case shown="True" w422 {
          tunnel: w417 -> [w433 w436]
          tunnel: [w433 w438] -> w416
          tunnel: w414 -> [w432 _]
          tunnel: [w432 w443] -> w412
          tunnel: w413 -> [_ w434]
          tunnel: w421 -> [w431 w442]
          tunnel: [w431 w441] -> w420
          tunnel: w419 -> [w430 w440]
          tunnel: [w430 w439] -> w418
          tunnel: w415 -> [_ w435]
          frame False {
          }
          frame True {
            n204 = call "HH_GetSyncPeriod.vi"("error in (no error)"=w436, "devidx"=w435) -> ("error out"=w438:errorcluster, "period"=w437:dbl)  [unwired: 7 in, 1 out]
            n205 = Reciprocal(x=w437) -> (1/x=w444:dbl)
            n206 = To Long Integer(number=w444) -> (32bit integer=w443:i32)
            n207 = case shown="Default" w434 {
              selector: w434 -> [w445 _ _]
              tunnel: w443 -> [w448 w468 _]
              tunnel: w442 -> [w446 w471 w475]
              tunnel: [w447 w471 w475] -> w441
              tunnel: w440 -> [w452 w470 w474]
              tunnel: [w452 w469 w473] -> w439
              frame Default {
                n208 = Subtract(x=w448, y=w445) -> (x-y=w451:i32)
                n209 = Absolute Value(x=w451) -> (abs(x)=w449:i32)
                n210 = Not Equal To 0?(x=w449) -> (x != 0?=w450:bool)
                n211 = case shown="True" w450 {
                  tunnel: w449 -> [_ w461]
                  tunnel: [w453 w456] -> w447
                  tunnel: w446 -> [w453 w455]
                  tunnel: w445 -> [_ w454]
                  frame False {
                  }
                  frame True {
                    n212 = To Double Precision Float(number=w461) -> (double precision float=w460:dbl)
                    n213 = To Double Precision Float(number=w454) -> (double precision float=w462:dbl)
                    n214 = Divide(x=w460, y=w462) -> (x/y=w459:dbl)
                    n215 = Greater Or Equal?(x=w459, y=0.01) -> (x >= y?=w457:bool)
                    n216 = case shown="False" w457 {
                      tunnel: [w463 w466] -> w456
                      tunnel: w455 -> [w463 w464]
                      frame False {
                      }
                      frame True {
                        w465 = T10[] [enum."StopMeas"] items=["Idle", "Init", "SetInpChanEnable", "SetInpChanOffset", "SetInpChanTrg", "SetSyncDivider", "SetSyncTrg", "SetSyncOffset", "SetBinning", "SetHistoOffset", "SetHistoLen", "SetStopOvl", "SetBitShift", "SetHistoAcqTime", "GetRates", "StartMeas", "StopMeas", "AbortMeas", "GetResolution", "GetHisto", "ReadFiFo", "WriteStatus", "Resize", "EnableControls", "DisableControls", "Error", "Exit"]
                        n217 = One Button Dialog(message="Warning: Sync Rate has changed!\nTime Trace resolution has been changed accordingly.\nMeasurement is aborted.\n") -> ()  [unwired: 1 in, 1 out]
                        n218 = Build Array (concatenate)(w464, w465) -> (w466:T10[])
                      }
                    }
                  }
                }
              }
              frame -1 {
                n219 = Bundle By Name(cluster=w470, "SyncRateStart"=w468) -> (w469:T8)
              }
              frame -2 {
                n220 = Bundle By Name(cluster=w474, "SyncRateStart"=-1) -> (w473:T8)
              }
            }
          }
        }
        n221 = for {
          N: w428 -> [_]
          tunnel: w415 -> [w481]
          tunnel: [w478] -> w426 mode=indexing
          shift-right: [w480] -> w429
          shift-left: w416 -> [w482]
          tunnel: w424 -> [w477] mode=indexing
          i -> [w479]
          n222 = Unbundle By Name(w477) -> ("Enable"=w476:bool)
          n223 = case shown="True" w476 {
            tunnel: w482 -> [w483 w488]
            tunnel: w481 -> [_ w487]
            tunnel: [w483 w486] -> w480
            tunnel: w479 -> [_ w485]
            tunnel: [_ w484] -> w478
            frame False {
            }
            frame True {
              n224 = call "HH_GetCountRate.vi"("error in (no error)"=w488, "Channel"=w485, "devidx"=w487) -> ("error out"=w486:errorcluster, "rate"=w484:i32)  [unwired: 6 in, 1 out]
            }
          }
        }
        "CountRates" <- w426
        n225 = Format Into String(format string="Sync Rate: %d cps\n", w412) -> (resulting string=→"SyncRate":string)  [unwired: 2 in, 1 out]
        n226 = Bundle By Name(cluster=w418, "SyncRate"=w412) -> (w423:T8)
      }
      frame "StartMeas" {
        # "Starts the actual measurement by calling the driver function 'HH_StartMeas' and passing the acquisition time to it. Also the 'HH_DataProcThread' is initialized for a new measurement by putting the command 'Init' to the DataProcQ. The command 'ReadFiFo' is inserted to the UIThreads CmdQ (the shift register)."
        n227 = Bundle By Name(cluster=T7 {"Cmd"=enum."Proc", "nActual"=0, "Buffer"=[], "TickCount"=0, "Param"=0} ("MH_DataProcThread_QData"), "Cmd"=HH_DataProcThread_QCmds."Init") -> (w493:T7)
        n228 = Unbundle By Name(w491) -> ("DevIdx"=w500:i32, "AcqTime"=w496:i32)
        n229 = Enqueue Element(queue=w495, element=w493) -> ()  [unwired: 2 in, 3 out]
        n230 = Bundle By Name(cluster=w491, "SyncRateStart"=-2) -> (w490:T8)
        n231 = call "HH_StartMeas.vi"("tacq"=w496, "devidx"=w500) -> ("error out"=w501:errorcluster)  [unwired: 8 in, 1 out]
        n232 = Build Array (concatenate)(w499, HH_UIThread_Cmds."ReadFiFo") -> (w498:T10[])
      }
      frame "StopMeas" {
        n233 = Unbundle By Name(w507) -> ("Run cont."=w502:bool, "DevIdx"=w508:i32)
        n234 = call "HH_StopMeas.vi"("devidx"=w508) -> ("error out"=w509:errorcluster)  [unwired: 9 in, 1 out]
        n235 = case shown="False" w502 {
          tunnel: w507 -> [w513 w515]
          tunnel: [w512 w515] -> w506
          tunnel: [w510 w514] -> w505
          frame False {
            w510 = T10[] [enum."ReadFiFo"] items=["Idle", "Init", "SetInpChanEnable", "SetInpChanOffset", "SetInpChanTrg", "SetSyncDivider", "SetSyncTrg", "SetSyncOffset", "SetBinning", "SetHistoOffset", "SetHistoLen", "SetStopOvl", "SetBitShift", "SetHistoAcqTime", "GetRates", "StartMeas", "StopMeas", "AbortMeas", "GetResolution", "GetHisto", "ReadFiFo", "WriteStatus", "Resize", "EnableControls", "DisableControls", "Error", "Exit"]
            w511 = FALSE ("StartMeas")
            n236 = Bundle By Name(cluster=w513, "StartMeas"=w511) -> (w512:T8)
            n237 = local write "Start"(w511) -> ()
          }
          frame True {
            w514 = T10[] [enum."ReadFiFo", enum."StartMeas"] items=["Idle", "Init", "SetInpChanEnable", "SetInpChanOffset", "SetInpChanTrg", "SetSyncDivider", "SetSyncTrg", "SetSyncOffset", "SetBinning", "SetHistoOffset", "SetHistoLen", "SetStopOvl", "SetBitShift", "SetHistoAcqTime", "GetRates", "StartMeas", "StopMeas", "AbortMeas", "GetResolution", "GetHisto", "ReadFiFo", "WriteStatus", "Resize", "EnableControls", "DisableControls", "Error", "Exit"]
          }
        }
        n238 = Build Array (concatenate)(w504, w505) -> (w503:T10[])
      }
      frame "AbortMeas" {
        w517 = FALSE ("StartMeas")
        n239 = Unbundle By Name(w519) -> ("DevIdx"=w520:i32)
        n240 = call "HH_StopMeas.vi"("devidx"=w520) -> ("error out"=w521:errorcluster)  [unwired: 9 in, 1 out]
        n241 = Bundle By Name(cluster=w519, "StartMeas"=w517) -> (w518:T8)
        n242 = local write "Start"(w517) -> ()
      }
      frame "GetResolution" {
        # "Resolution in ns"
        # "Gets resolution in ps"
        # "Resolution is saved in UIThread Data cluster in ns"
        n243 = Unbundle By Name(w530) -> ("DevIdx"=w532:i32)
        n244 = call "HH_GetResolution.vi"("devidx"=w532) -> ("error out"=w531:errorcluster, "resolution"=w528:dbl)  [unwired: 8 in, 1 out]
        n245 = Divide(x=w528, y=1000.0) -> (x/y=w524:dbl)
        n246 = Bundle By Name(cluster=w530, "Resolution"=w524) -> (w529:T8)
        n247 = Bundle By Name(cluster=T5 {"Histos"=[], "Cmd"=enum."_none_", "TimeTrace"=[], "Bin"=0, "Total bin"=0, "Status"="", "Resol"=0.0, "DeltaT"=0.0, "nChannels"=0} ("MH_GUIThread_QData"), "Resol"=w524, "Cmd"=HH_VisThread_QCmds."Resol") -> (w522:T5)
        n248 = Enqueue Element(queue=w526, element=w522) -> ()  [unwired: 2 in, 3 out]
      }
      frame "ReadFiFo" {
        w542 = 2  # FLAG_FIFOFULL
        # "Reads photon records from HW and transferes them to DataProcThread via Queue."
        n249 = Unbundle By Name(w544) -> ("DevIdx"=w538:i32)
        n250 = call "HH_GetFlags.vi"("devidx"=w538) -> ("error out"=w540:errorcluster, "flags"=w541:i32)  [unwired: 8 in, 1 out]
        n251 = And(x=w541, y=w542) -> (x .and. y?=w543:i32)
        n252 = Not Equal To 0?(x=w543) -> (x != 0?=w537:bool)
        "OverRun" <- w537
        n253 = case shown="False" w537 {
          tunnel: w540 -> [w554 w557]
          tunnel: [w553 w557] -> w539
          tunnel: w538 -> [w546 _]
          tunnel: w536 -> [w552 _]
          tunnel: w535 -> [w551 _]
          tunnel: [w551 w555] -> w534
          frame False {
            n254 = call "HH_ReadFiFo.vi"("error in (no error)"=w554, "devidx"=w546) -> ("error out"=w553:errorcluster, "nactual"=w545:i32, "buffer"=w549:u32[])  [unwired: 6 in, 1 out]
            n255 = Bundle By Name(cluster=T7 {"Cmd"=enum."Proc", "nActual"=0, "Buffer"=[], "TickCount"=0, "Param"=0} ("MH_DataProcThread_QData"), "Buffer"=w549, "nActual"=w545, "Cmd"=HH_DataProcThread_QCmds."Proc") -> (w547:T7)
            n256 = Enqueue Element(queue=w552, element=w547) -> ()  [unwired: 2 in, 3 out]
          }
          frame True {
            n257 = Build Array(HH_UIThread_Cmds."AbortMeas") -> (w555:T10[])
          }
        }
      }
      frame "WriteStatus" {
        n258 = Unbundle By Name(w559) -> ("Status"=→"Status":string)
      }
      frame "Resize" {
        n259 = property on="Pane 3" class="Pane"() -> ("Width"=w566:u32)  [unwired: 2 in, 2 out]
        n260 = Subtract(x=w566, y=i16 100 ("b")) -> (x-y=w572:u32)
        n261 = Unbundle By Name(w561) -> ("Init Info.nchannels"=w569:i32)
        n262 = Quotient & Remainder(x=w572, y=i16 99 ("m")) -> (floor(x/y)=w571:u32)  [unwired: 1 out]
        n263 = In Range and Coerce(upper limit=w569, x=w571, lower limit=4) -> (coerced(x)=w570:u32)  [unwired: 1 out]
        n264 = Equal?(x=w569, y=w570) -> (x = y?=w568:bool)
        n265 = Not(x=w568) -> (.not. x?=w567:bool)
        n266 = property on="Channels" class="Arr (strict)"("HorizScroll"=w567, "Number of Columns"=w570, "Index Values"=u32[] [0]) -> ()  [unwired: 2 in, 2 out]
      }
      frame "EnableControls" {
        n267 = property class="VI"() -> ("Panel"=w577:refnum<vi>)  [unwired: 2 in, 2 out]
        n268 = property class="Pnl"(reference=w577) -> ("Controls[]"=w576:refnum<vi>[])  [unwired: 1 in, 2 out]
        n269 = property class="Pnl"(reference=w577) -> ("Decos[]"=w578:refnum<vi>[])  [unwired: 1 in, 2 out]
        n270 = for {
          tunnel: w578 -> [w582] mode=indexing
          tunnel: TRUE -> [w581]
          n271 = property class="Decor"(reference=w582, "Visible"=w581) -> ()  [unwired: 1 in, 2 out]
        }
        n272 = for {
          tunnel: w576 -> [w585] mode=indexing
          tunnel: T11."Enabled" ("Disabled") -> [w584]
          tunnel: [w583] -> _
          n273 = property class="Ctl"(reference=w585, "DisabledEnum"=w584) -> (error out=w583:errorcluster)  [unwired: 1 in, 1 out]
        }
      }
      frame "DisableControls" {
        n274 = property class="VI"() -> ("Panel"=w589:refnum<vi>)  [unwired: 2 in, 2 out]
        n275 = property class="Pnl"(reference=w589) -> ("Controls[]"=w588:refnum<vi>[])  [unwired: 1 in, 2 out]
        n276 = property class="Pnl"(reference=w589) -> ("Decos[]"=w590:refnum<vi>[])  [unwired: 1 in, 2 out]
        n277 = for {
          tunnel: w590 -> [w594] mode=indexing
          tunnel: FALSE -> [w593]
          n278 = property class="Decor"(reference=w594, "Visible"=w593) -> ()  [unwired: 1 in, 2 out]
        }
        n279 = for {
          tunnel: w588 -> [w597] mode=indexing
          tunnel: T11."Disabled and Grayed Out" ("Disabled") -> [w596]
          tunnel: [w595] -> _
          n280 = property class="Ctl"(reference=w597, "DisabledEnum"=w596) -> (error out=w595:errorcluster)  [unwired: 1 in, 1 out]
        }
      }
      frame "Error" {
        w598 = T10[] [enum."Exit"] items=["Idle", "Init", "SetInpChanEnable", "SetInpChanOffset", "SetInpChanTrg", "SetSyncDivider", "SetSyncTrg", "SetSyncOffset", "SetBinning", "SetHistoOffset", "SetHistoLen", "SetStopOvl", "SetBitShift", "SetHistoAcqTime", "GetRates", "StartMeas", "StopMeas", "AbortMeas", "GetResolution", "GetHisto", "ReadFiFo", "WriteStatus", "Resize", "EnableControls", "DisableControls", "Error", "Exit"]
        w601 = T14 1 items=["no dialog", "OK message", "continue or stop message", "OK message + warnings", "continue/stop + warnings"] ("type of dialog (OK msg:1)")
        # "Error case: If an error occures the user is informed and the programm terminates. Add your own code to handle error events (e.g. exception lists, etc.)"
        n281 = call <vilib>:"Simple Error Handler.vi"("type of dialog (OK msg:1)"=w601, "error in (no error)"=w600) -> ()  [unwired: 3 in, 5 out]
      }
      frame "Exit" {
        n282 = Release Queue(queue=w603) -> ()  [unwired: 2 in, 3 out]
        n283 = Release Queue(queue=w602) -> ()  [unwired: 2 in, 3 out]
        n284 = Unbundle By Name(w607) -> ("DevIdx"=w606:i32)
        n285 = call "HH_CloseDevice.vi"("devidx"=w606) -> ("error out"=w605:errorcluster)  [unwired: 9 in, 1 out]
      }
    }
    n286 = call "HH_EnQError.vi"("error in (no error)"=w24, "Cmds_in"=w22) -> ("error out"=w23:errorcluster, "Cmds_out"=w21:T10[])  [unwired: 8 in]
  }
  n287 = call "HH_DataProcThread.vi"("HH_VisThread_QRef"=w7, "HH_DataProcThread_QRef"=w1) -> ()  [unwired: 10 in]
  n288 = while {
    tunnel: w7 -> [w616]
    shift-right: [w612] -> _
    shift-left: T4 {"Resol"=0.0, "DeltaT"=0.0, "NumChannels"=0} -> [w613]
    tunnel: w1 -> [w611]
    stop <- w609 stop-if-true
    # "VisualizationThread"
    n289 = Dequeue Element(queue=w616, timeout in ms (-1)=100) -> (element=w614:T5, error out=w609:errorcluster)  [unwired: 1 in, 2 out]
    n290 = Unbundle By Name(w614) -> ("Cmd"=w615:T6)
    n291 = case shown="\"DeltaT\"" w615 {
      tunnel: w614 -> [_ w629 w631 w643 w651 w655 w659]
      tunnel: w613 -> [w619 w627 w633 w635 w650 w654 w658]
      tunnel: [w619 w627 w632 w635 w650 w653 w657] -> w612
      tunnel: w611 -> [w618 _ _ _ w647 _ _]
      tunnel: w609 -> [w617 _ _ _ _ _ _]
      frame "_none_", Default {
        n292 = case shown="No Error" w617 {
          tunnel: w618 -> [w623 _]
          frame No Error {
            n293 = Get Queue Status(queue=w623) -> (# elements in queue=w621:i32)  [unwired: 2 in, 7 out]
            n294 = Format Into String(format string="Elements in Q: %d", w621) -> (resulting string=w620:string)  [unwired: 2 in, 1 out]
            n295 = local write "Status"(w620) -> ()
          }
          frame Error {
          }
        }
      }
      frame "Histo" {
        n296 = Unbundle By Name(w629) -> ("Histos"=w624:u32[][])
        n297 = Unbundle By Name(w627) -> ("Resol"=w626:dbl)
        n298 = Bundle(0.0, "Resol"=w626, "Histos"=w624) -> (→"HistoGraph":cluster{dbl, "Resol":dbl, "Histos":u32[][]})  [unwired: 1 in]
      }
      frame "nChannels" {
        n299 = Unbundle By Name(w631) -> ("nChannels"=w630:i32)
        n300 = Bundle By Name(cluster=w633, "NumChannels"=w630) -> (w632:T4)
      }
      frame "TTrace" {
        n301 = Unbundle By Name(w643) -> ("Total bin"=w642:u64, "Bin"=w641:i32, "TimeTrace"=w640:u32[][])
        n302 = Unbundle By Name(w635) -> ("DeltaT"=w634:dbl)
        n303 = call "HH_TTraceToGraph.vi"("DeltaT"=w634, "TimeTrace"=w640, "Bin"=w641, "Total bin"=w642) -> ("TimeTrace_out"=w637:u32[][], "dt"=w638:dbl, "T0"=w639:dbl)  [unwired: 5 in]
        n304 = Bundle("T0"=w639, "dt"=w638, "TimeTrace_out"=w637) -> (→"TTraceGraph":T15)  [unwired: 1 in]
      }
      frame "Status" {
        n305 = Unbundle By Name(w651) -> ("Status"=w648:string)
        n306 = Get Queue Status(queue=w647) -> (# elements in queue=w646:i32)  [unwired: 2 in, 7 out]
        n307 = Format Into String(format string="\t\tElements in Q: %d", w646) -> (resulting string=w644:string)  [unwired: 2 in, 1 out]
        n308 = Concatenate Strings(w648, w644) -> (w649:string)
        n309 = local write "Status"(w649) -> ()
      }
      frame "DeltaT" {
        n310 = Unbundle By Name(w655) -> ("DeltaT"=w652:dbl)
        n311 = Bundle By Name(cluster=w654, "DeltaT"=w652) -> (w653:T4)
      }
      frame "Resol" {
        n312 = Unbundle By Name(w659) -> ("Resol"=w656:dbl)
        n313 = Bundle By Name(cluster=w658, "Resol"=w656) -> (w657:T4)
      }
    }
  }
